vi "error_check_shutdown_freq_sweep_agilent.vi"(8 "?":T1=enum."Shutdown", 11 "Boolean":bool) -> (3 "?":T1=enum."Shutdown")   [LabVIEW 2017]
uses:
  controls/State.ctl
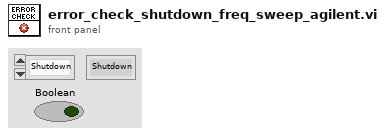
[diagram p1: front panel]
types:
  T1 = typedef "State.ctl" = enum16{"Init", "Idle", "Configuring", "Sweeping to ref", "Measuring ref", "Sweeping to H", "Measuring H", "Sweeping down", "Shutdown"}
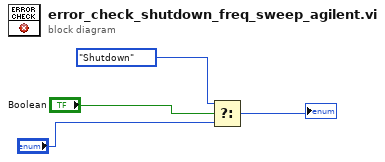
[diagram p0: block diagram]
diagram:
  n1 = Select(t=State."Shutdown", s="Boolean", f="?") -> (s? t:f=→"?":T1)
